vi "(SubVI) Acquire ADC and DAC Rate of Stage_YCC.vi"() -> (2 "adcfreq-read (ms)":dbl, 3 "adcfreq-read (Hz)":dbl, 4 "dacfreq-write (ms)":dbl, 5 "dacfreq-write (Hz)":dbl)   [LabVIEW 2014]
uses:
  Main-Stage-PI/(Global) Current handle and LaserPower_YCC.vi
  MCL-dll-Labview 32-bit/Madlib.dll
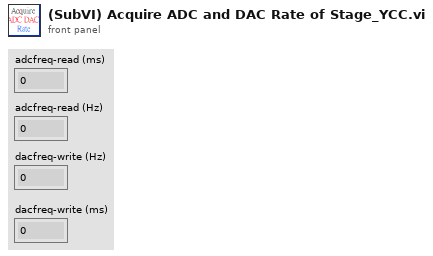
[diagram p1: front panel]
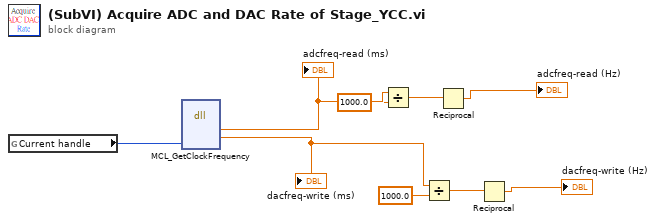
[diagram p0: block diagram]
diagram:
  n1 = global read "(Global) Current handle and LaserPower_YCC.vi" "Current handle"() -> (w9:i32)
  n2 = dll-call lib="C:/Users/hwlab/OneDrive - g.ntu.edu.tw/OT/YCC's OT-PI/Main-Stage-Based/SubVI-Stage-Based/MCL-dll-Labview 32-bit/Madlib.dll" fn="MCL_GetClockFrequency" label="MCL_SingleWriteN"("handle"=w9) -> ("adcfreq (ms)"=w8:dbl, "dacfreq (ms)"=w2:dbl)  [unwired: 7 in, 2 out]
  "adcfreq-read (ms)" <- w8
  "dacfreq-write (ms)" <- w2
  n3 = Divide(x=w8, y=1000.0) -> (x/y=w6:dbl)
  n4 = Divide(x=w2, y=1000.0) -> (x/y=w3:dbl)
  n5 = Reciprocal(x=w6) -> (1/x=→"adcfreq-read (Hz)":dbl)
  n6 = Reciprocal(x=w3) -> (1/x=→"dacfreq-write (Hz)":dbl)
